vi "Chart[Template].SetDependencies.vi"(8 "error in (no error)":errorcluster, 10 "Dependencies":T1, 11 "DisplayWaveforms":refnum<class "DisplayWaveforms.lvclass">) -> (0 "error out":errorcluster, 3 "DisplayWaveforms out":refnum<class "DisplayWaveforms.lvclass">)   [LabVIEW 2018, in "DisplayWaveform.lvlib" / "DisplayWaveforms.lvclass"]
doc: "---------------------------------------------------------------\nJKI State Machine Objects™\nhttp://jki.net/state-machine-objects/\nCopyright (C) 2005-2015, JKI <info@jki.net>\nALL RIGHTS RESERVEDJKI State Machine Objects (SMO) 1.0.0.5\nJKI - JKI\nCopyright (c) 2016, JKI"
uses:
  DisplayWaveforms.lvclass
  Typedefs/Dependencies--Cluster.ctl
panel:
  # "For instructions on how to use the JKI State Machine Objects, examples and video tutorials, visit:\nhttp://jki.net/state-machine-objects/\n\nJKI State Machine Objects™\nhttp://jki.net/state-machine-objects/\nCopyright (C) 2005-2015, JKI <info@jki.net>\nALL RIGHTS RESERVED"
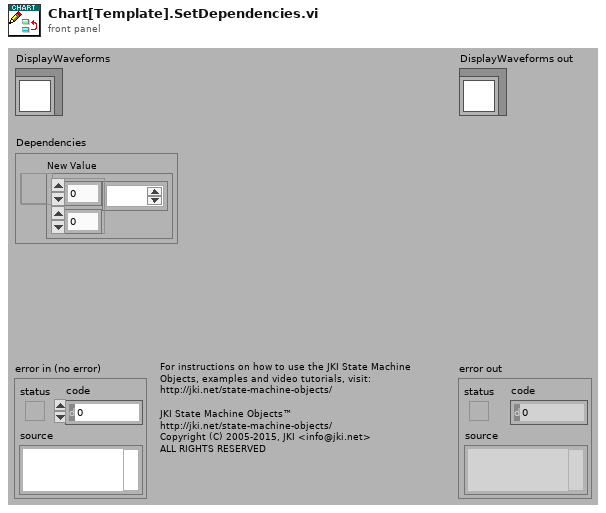
[diagram p1: front panel]
types:
  T1 = typedef "DisplayWaveform.lvlib/DisplayWaveforms.lvclass/Dependencies--Cluster.ctl" = cluster{"New Value":refnum<user-event>}
  T2 = typedef "DisplayWaveform.lvlib/DisplayWaveforms.lvclass/PrivateData--Ref.ctl" = refnum<data-value>
  T3 = typedef "DisplayWaveform.lvlib/DisplayWaveforms.lvclass/PrivateData--Cluster.ctl" = cluster{"Public Events":T4, "Protected Events":T5, "Data":string, "Dependencies":T1}
  T4 = typedef "DisplayWaveform.lvlib/DisplayWaveforms.lvclass/PublicEvents--Cluster.ctl" = cluster{"Chart Cleared":refnum<user-event>, "Chart Exported":refnum<user-event>, "ChartParams Set":refnum<user-event>}
  T5 = typedef "DisplayWaveform.lvlib/DisplayWaveforms.lvclass/ProtectedEvents--Cluster.ctl" = cluster{"Clear Chart":refnum<user-event>, "Pause Chart":refnum<user-event>, "Update Chart":refnum<user-event>, "Export Chart":refnum<user-event>, "Set ChartParams":refnum<user-event>}
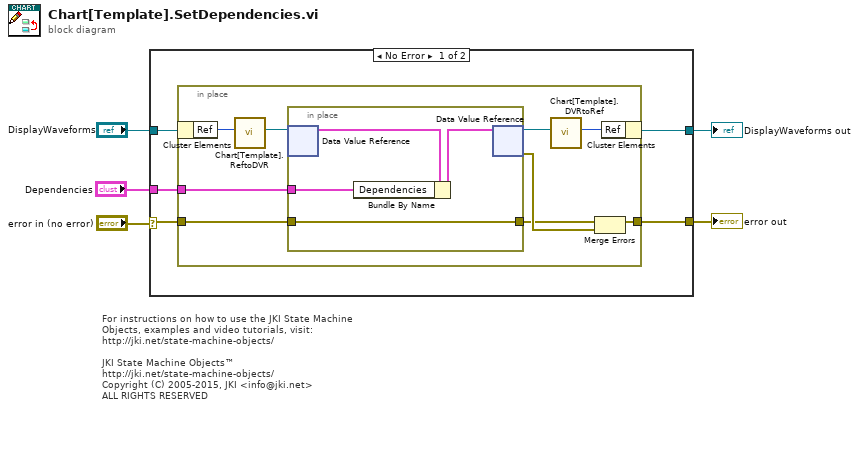
[diagram p0: block diagram]
diagram:
  # "For instructions on how to use the JKI State Machine Objects, examples and video tutorials, visit:\nhttp://jki.net/state-machine-objects/\n\nJKI State Machine Objects™\nhttp://jki.net/state-machine-objects/\nCopyright (C) 2005-2015, JKI <info@jki.net>\nALL RIGHTS RESERVED"
  n1 = case shown="No Error" "error in (no error)" {
    selector: "error in (no error)" -> [w9 w24]
    tunnel: "DisplayWaveforms" -> [w10 w25]
    tunnel: [w8 w24] -> w4
    tunnel: [w7 w25] -> w3
    tunnel: "Dependencies" -> [w6 _]
    frame No Error {
      n2 = in-place {
        in-place-border: w9 -> [w19]
        in-place-border: [w16] -> w8
        in-place-border: w6 -> [w11]
        n3 = in-place-cluster #1(w10) -> ("Ref"=w15:u32)
        n4 = call "Chart[Template].ReftoDVR.vi"("Ref"=w15) -> ("Ref"=w14:T2)  [unwired: 10 in]
        n5 = in-place {
          in-place-border: w19 -> [w23]
          in-place-border: [w23] -> w17
          in-place-border: w11 -> [w20]
          n6 = in-place-dvr #2(w14) -> (w22:T3)  [unwired: 1 out]
          n7 = Bundle By Name(cluster=w22, "Dependencies"=w20) -> (w21:T3)
          n8 = in-place-dvr #2(w21) -> (w13:T2, w18:errorcluster)
        }
        n9 = call "Chart[Template].DVRtoRef.vi"("Ref"=w13) -> ("Ref"=w12:u32)  [unwired: 10 in]
        n10 = Merge Errors(w17, w18) -> (w16:errorcluster)
        n11 = in-place-cluster #1("Ref"=w12) -> (w7:refnum<class "DisplayWaveforms.lvclass">)
      }
    }
    frame Error {
    }
  }
  "error out" <- w4
  "DisplayWaveforms out" <- w3
